vi "LaserDiodeInit.vi"(6 "resource name":refnum<visa-resource-name>) -> (0 "Diode Driver Error":errorcluster caption="error in (no error)" {"code" format="%.0x"}, 1 "Temperature":dbl, 2 "TEC Output":bool, 3 "resource out":refnum<visa-resource-name> caption="resource name", 4 "LD Output":bool, 5 "Serial Number":string)   [LabVIEW 2019]
panel:
  out "Diode Driver COM":refnum<visa-resource-name>="USB0::0x1313::0x804F::M00549740::INSTR"
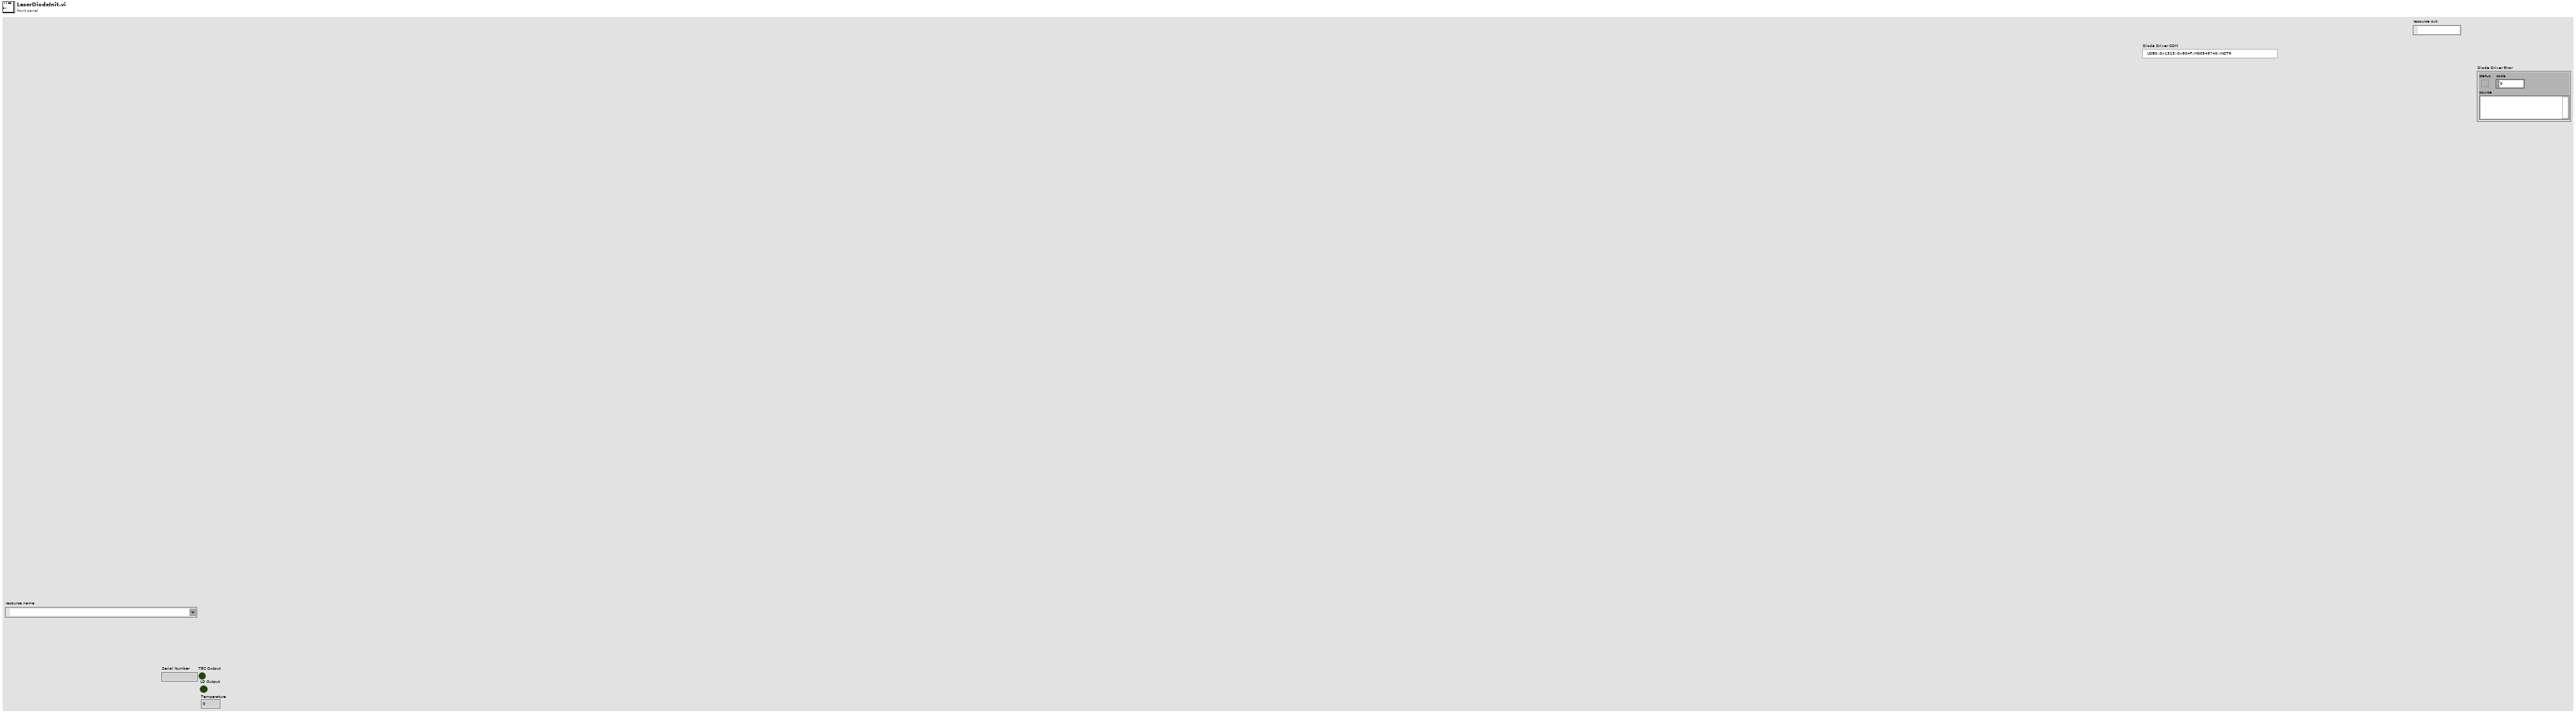
[diagram p1: front panel]
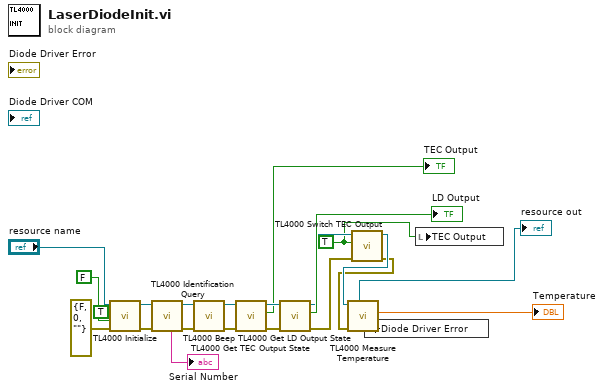
[diagram p0: block diagram]
diagram:
  w1 = TRUE ("TEC Output (Off)")
  n1 = call <instrlib>:"TL4000 Initialize.vi"("error in (no error)"=errorcluster {"status"=FALSE, "code"=0, "source"=""}, "Reset Device (Reset Device)"=FALSE ("ID Query (Do Query)"), "ID Query (Do Query)"=TRUE, "resource name"="resource name") -> ("error out"=w17:errorcluster, "instrument handle out"=w16:refnum<visa-resource-name>)  [unwired: 6 in]
  n2 = call <instrlib>:"TL4000 Identification Query.vi"("error in (no error)"=w17, "instrument handle"=w16) -> ("error out"=w20:errorcluster, "instrument handle out"=w18:refnum<visa-resource-name>, "Serial Number"=→"Serial Number":string)  [unwired: 4 in, 3 out]
  n3 = call <instrlib>:"TL4000 Beep.vi"("error in (no error)"=w20, "instrument handle"=w18) -> ("error out"=w21:errorcluster, "instrument handle out"=w19:refnum<visa-resource-name>)  [unwired: 8 in]
  n4 = call <instrlib>:"TL4000 Get TEC Output State.vi"("error in (no error)"=w21, "instrument handle"=w19) -> ("error out"=w14:errorcluster, "TEC Output"=→"TEC Output":bool, "instrument handle out"=w15:refnum<visa-resource-name>)  [unwired: 7 in]
  n5 = call <instrlib>:"TL4000 Get LD Output State.vi"("error in (no error)"=w14, "instrument handle"=w15) -> ("error out"=w3:errorcluster, "LD Output"=→"LD Output":bool, "instrument handle out"=w4:refnum<visa-resource-name>)  [unwired: 7 in]
  n6 = call <instrlib>:"TL4000 Switch TEC Output.vi"("error in (no error)"=w3, "TEC Output (Off)"=w1, "instrument handle"=w4) -> ("error out"=w2:errorcluster, "instrument handle out"=w5:refnum<visa-resource-name>)  [unwired: 7 in]
  n7 = call <instrlib>:"TL4000 Measure Temperature.vi"("error in (no error)"=w2, "instrument handle"=w5) -> ("error out"=w23:errorcluster, "Temperature"=→"Temperature":dbl, "instrument handle out"=→"resource out":refnum<visa-resource-name>)  [unwired: 7 in]
  n8 = local write "Diode Driver Error"(w23) -> ()
  n9 = local write "TEC Output"(w1) -> ()
